vi "DistanceFunction.vi"(4 "Condition Driver":bool, 6 "Position (real coords)":cluster{dbl, dbl, "Z":dbl}, 9 "Current Spot Number":refnum<vi>, 10 "Spot Checker":refnum<vi>, 11 "Spot Number Being Checked":refnum<vi>) -> (2 "Distance":dbl)   [LabVIEW 2015]
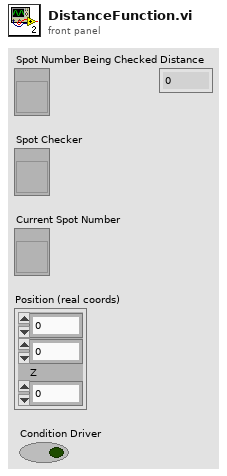
[diagram p1: front panel]
types:
  T1 = typedef "spot.ctl" = cluster{"Position":cluster{"x":dbl, "y":dbl, "z":dbl}, "Intensity":dbl, "Vortex Charge":i8, "Phase":dbl, "NA Position":cluster{"x":dbl, "y":dbl, "r":dbl}, "Line Trapping":T2, "Amplitude Correction":dbl}
  T2 = typedef "line_trapping.ctl" = cluster{"Vector":cluster{"x":dbl, "y":dbl, "z":dbl}, "Phase Gradient":dbl}
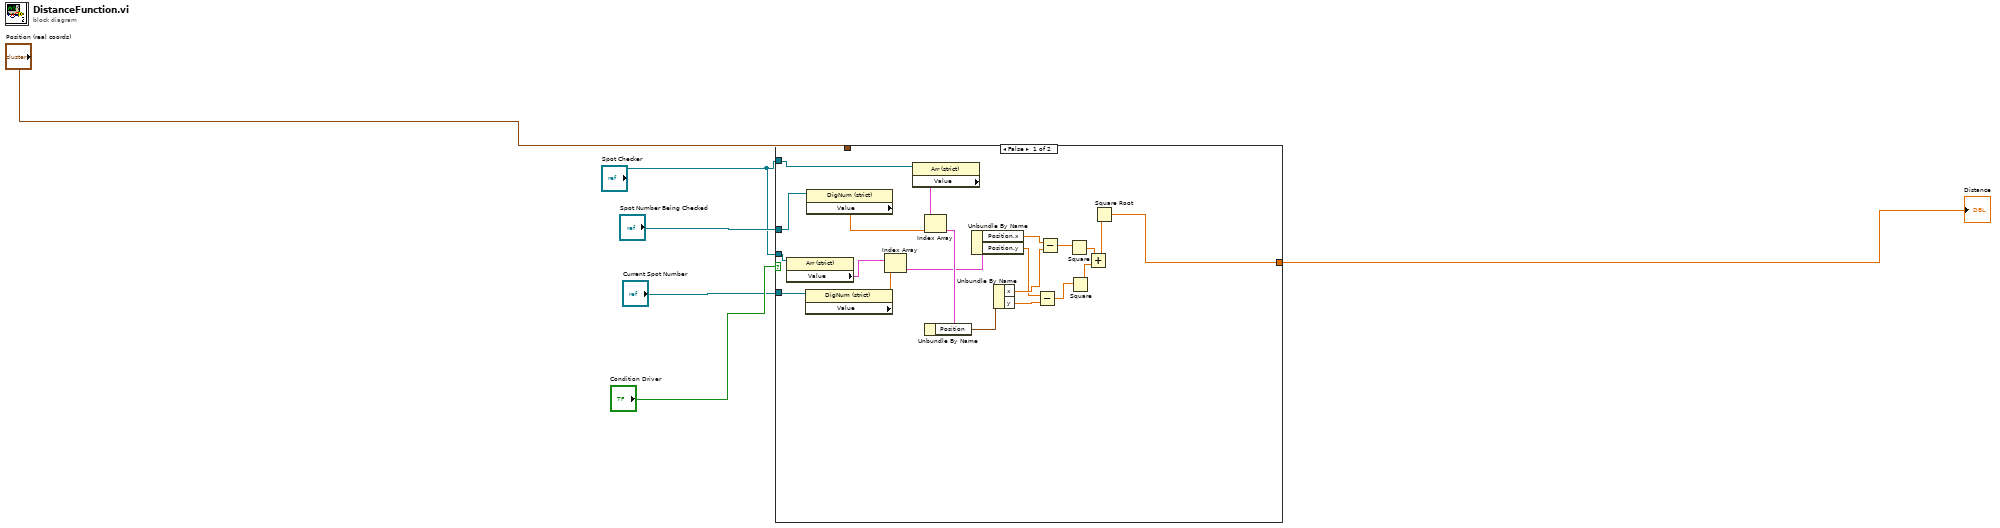
[diagram p0: block diagram]
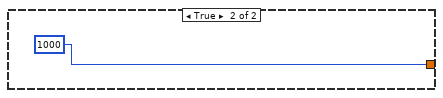
[diagram p2: hidden frame]
diagram:
  n1 = case shown="False" "Condition Driver" {
    tunnel: [w16 1000] -> w4
    tunnel: "Position (real coords)" -> [_ _]
    tunnel: "Spot Number Being Checked" -> [w10 _]
    tunnel: "Spot Checker" -> [w9 _]
    tunnel: "Spot Checker" -> [w8 _]
    tunnel: "Current Spot Number" -> [w7 _]
    frame False {
      n2 = property class="Arr (strict)"(reference=w8) -> ("Value"=w15:T1[])  [unwired: 1 in, 2 out]
      n3 = property class="DigNum (strict)"(reference=w7) -> ("Value"=w14:dbl)  [unwired: 1 in, 2 out]
      n4 = property class="DigNum (strict)"(reference=w10) -> ("Value"=w18:dbl)  [unwired: 1 in, 2 out]
      n5 = Index Array(array=w15, index=w14) -> (element=w13:T1)
      n6 = property class="Arr (strict)"(reference=w9) -> ("Value"=w17:T1[])  [unwired: 1 in, 2 out]
      n7 = Index Array(array=w17, index=w18) -> (element=w27:T1)
      n8 = Unbundle By Name(w27) -> ("Position"=w26:cluster{"x":dbl, "y":dbl, "z":dbl})
      n9 = Unbundle By Name(w13) -> ("Position.x"=w12:dbl, "Position.y"=w11:dbl)
      n10 = Unbundle By Name(w26) -> ("x"=w25:dbl, "y"=w24:dbl)
      n11 = Subtract(x=w11, y=w24) -> (x-y=w22:dbl)
      n12 = Subtract(x=w12, y=w25) -> (x-y=w23:dbl)
      n13 = Square(x=w23) -> (x^2=w21:dbl)
      n14 = Square(x=w22) -> (x^2=w20:dbl)
      n15 = Add(x=w21, y=w20) -> (x+y=w19:dbl)
      n16 = Square Root(x=w19) -> (sqrt(x)=w16:dbl)
    }
    frame True {
    }
  }
  "Distance" <- w4
